vi "decode double.vi"(11 "byte array in":u8[](array[numeric]) format="%.0b") -> (2 "double":dbl, 3 "byte array out":u8[](array[numeric]))   [LabVIEW 2013, in "protocol buffers encoder.lvlib"]
uses:
  protocol buffers encoder.lvlib
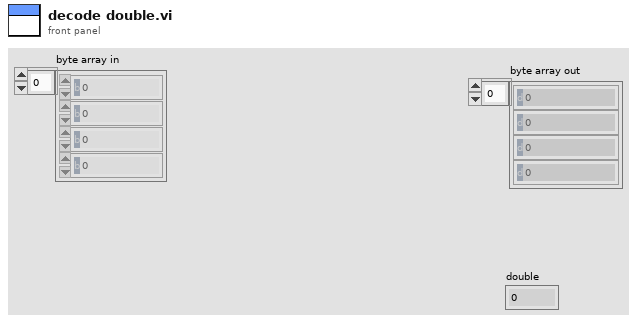
[diagram p1: front panel]
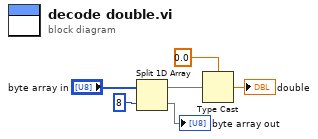
[diagram p0: block diagram]
diagram:
  n1 = Split 1D Array(array="byte array in", index=8) -> (first subarray=w3:u8[], second subarray=→"byte array out":u8[])
  n2 = Type Cast(type=0.0, x=w3) -> (*(type *) &x=→"double":dbl)
